vi "run_python_script_2_demoinfocom.vi"(9 "Rate of CR bits":u32, 10 "Number of Observations":u32) -> (1 "Secret Key KB":u8[](array[numeric]), 2 "Secret Key KA":u8[](array[numeric]))   [LabVIEW 2021]
panel:
  out "Size of Parity in bytes":u8[](array[numeric])
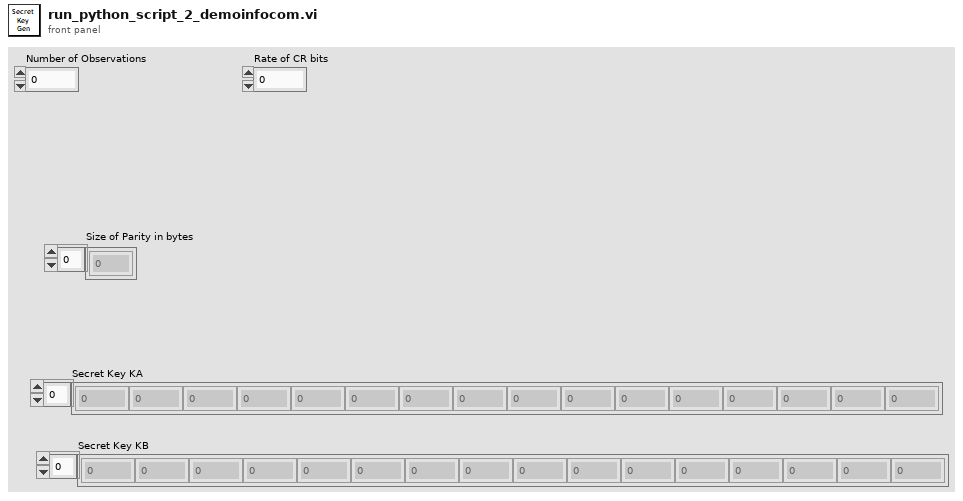
[diagram p1: front panel]
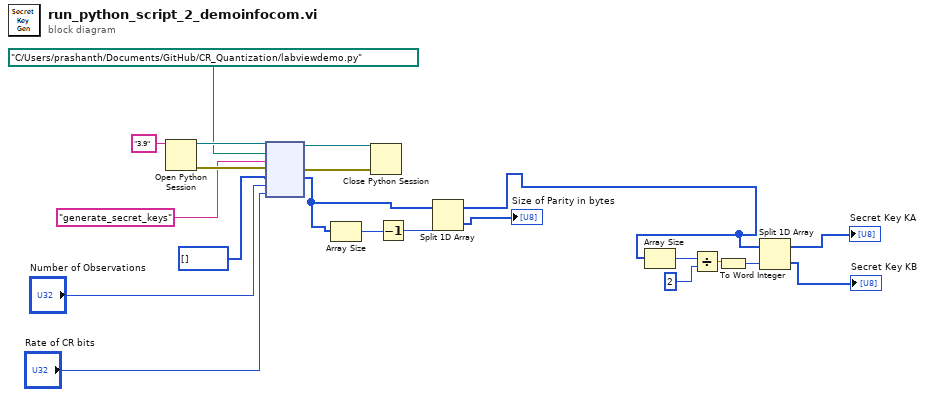
[diagram p0: block diagram]
diagram:
  n1 = Open Python Session(python version="3.9" ("Python version")) -> (session out=w21:refnum<k35>, error out=w19:errorcluster)  [unwired: 2 in]
  n2 = node ("Python Node")(w21, path "C:/Users/prashanth/Documents/GitHub/CR_Quantization/labviewdemo.py" ("module path"), "generate_secret_keys" ("function name"), w19, u8[] [], "Number of Observations", "Rate of CR bits") -> (w20:refnum<k35>, w18:errorcluster, w4:u8[])  [unwired: 2 in, 2 out]
  n3 = Array Size(array=w4) -> (size(s)=w6:i32)
  n4 = Close Python Session(session in=w20, error in=w18) -> ()  [unwired: 1 out]
  n5 = Decrement(x=w6) -> (x-1=w7:i32)
  n6 = Split 1D Array(array=w4, index=w7) -> (first subarray=w3:u8[], second subarray=→"Size of Parity in bytes":u8[])
  n7 = Array Size(array=w3) -> (size(s)=w13:i32)
  n8 = Divide(x=w13, y=2) -> (x/y=w11:dbl)
  n9 = To Word Integer(number=w11) -> (16bit integer=w10:i16)
  n10 = Split 1D Array(array=w3, index=w10) -> (first subarray=→"Secret Key KA":u8[], second subarray=→"Secret Key KB":u8[])
